vi "Basic Test Compile 2, Proof of Concept.vi"() -> ()   [LabVIEW 2009]
uses:
  Motor Control Global.vi
  <vilib>/Platform/TimedLoop/XDataNode/XDataNode.xnode
  <vilib>/Platform/TimedLoop/XDataNode/loadlvalarms.vi
  <vilib>/Platform/TimedLoop/XDataNode/timing_clust.ctl
  <vilib>/Platform/TimedLoop/XDataNode/nitl_modes.ctl
  <vilib>/Platform/TimedLoop/XDataNode/wakeup.ctl
  <vilib>/Platform/TimedLoop/XDataNode/XDNodeRunTimeDep.lvlib
panel:
  in  "Input A 2":fxp<+/-,18,1>
  out "13 Timed out":bool
  out "Timed out":bool
  out "12 Timed out":bool
  out "Tick Count Differencce":u32
  out "Tick Count(Ticks) 2":u32 caption="Tick Count(Ticks)"
  out "Tick Count(Ticks)":u32
  in  "Single Cycle":bool
  out "Multiplication Result":fxp<+/-,18,1> format="%.18g"
  out "i 3":i32
  out "i 2":i32
  out "i 1":i32
  out "in wait":bool=TRUE
  in  "Restart":bool
  in  "Input F":fxp<+/-,18,1>
  in  "Input E":fxp<+/-,18,1>
  out "Multiplication Result 8 iterations of madness":fxp<+/-,18,1> format="%.18g"
  in  "Input D":fxp<+/-,18,1>
  in  "Input C":fxp<+/-,18,1>
  out "Multiplication Result C^2^15 * D^2^15":fxp<+/-,18,1> format="%.18g"
  in  "stop":bool
  out "Multiplication Result A^60*B":fxp<+/-,18,1> format="%.18g"
  in  "Input A":fxp<+/-,18,1>
  in  "Input B":fxp<+/-,18,1>
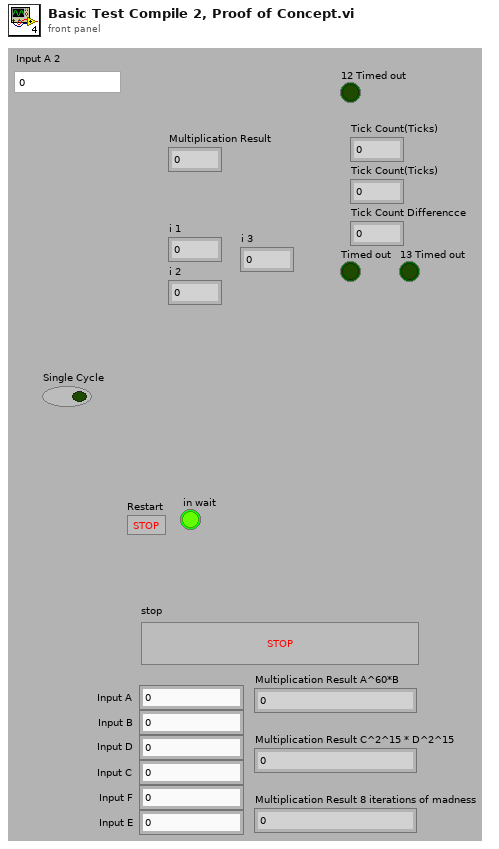
[diagram p1: front panel]
types:
  T1 = typedef "XDNodeRunTimeDep.lvlib/timing_clust.ctl" = cluster{"Expected End [f-1]":u64, "Actual End [f-1]":u64, "Finished Late? [f-1]":bool, "Expected End [i-1]":u64, "Actual End [i-1]":u64, "Finished Late? [i-1]":bool, "Expected Start [i]":u64, "Actual Start [i]":u64, "Expected Start [f]":u64, "Actual Start [f]":u64, "Source Name":string, "Structure Name":string, "Period":i64, "Deadline":i64, "Offset":i64, "Start":i64, "Priority":i32, "Timeout":i32, "Mode":T2, "Wakeup Reason":T3, "Error":errorcluster, "Source Type":string, "Secondary Source Type":string, "Global End Time":u64, "Global Start Time":u64, "Frame Duration":u64, "Iteration Duration":u64, "Assigned CPU":i32, "I/O Scan Engine Mode":u32}
  T2 = typedef "XDNodeRunTimeDep.lvlib/nitl_modes.ctl" = enum32{"No Change", "Process missed periods, maintain original phase", "Discard missed periods, maintain original phase", "Process missed periods, ignore original phase", "Discard missed periods, ignore original phase"}
  T3 = typedef "XDNodeRunTimeDep.lvlib/wakeup.ctl" = enum32{"Normal", "Aborted", "Asynchronous wakeup", "Timing source error", "Timed loop error", "Timeout"}
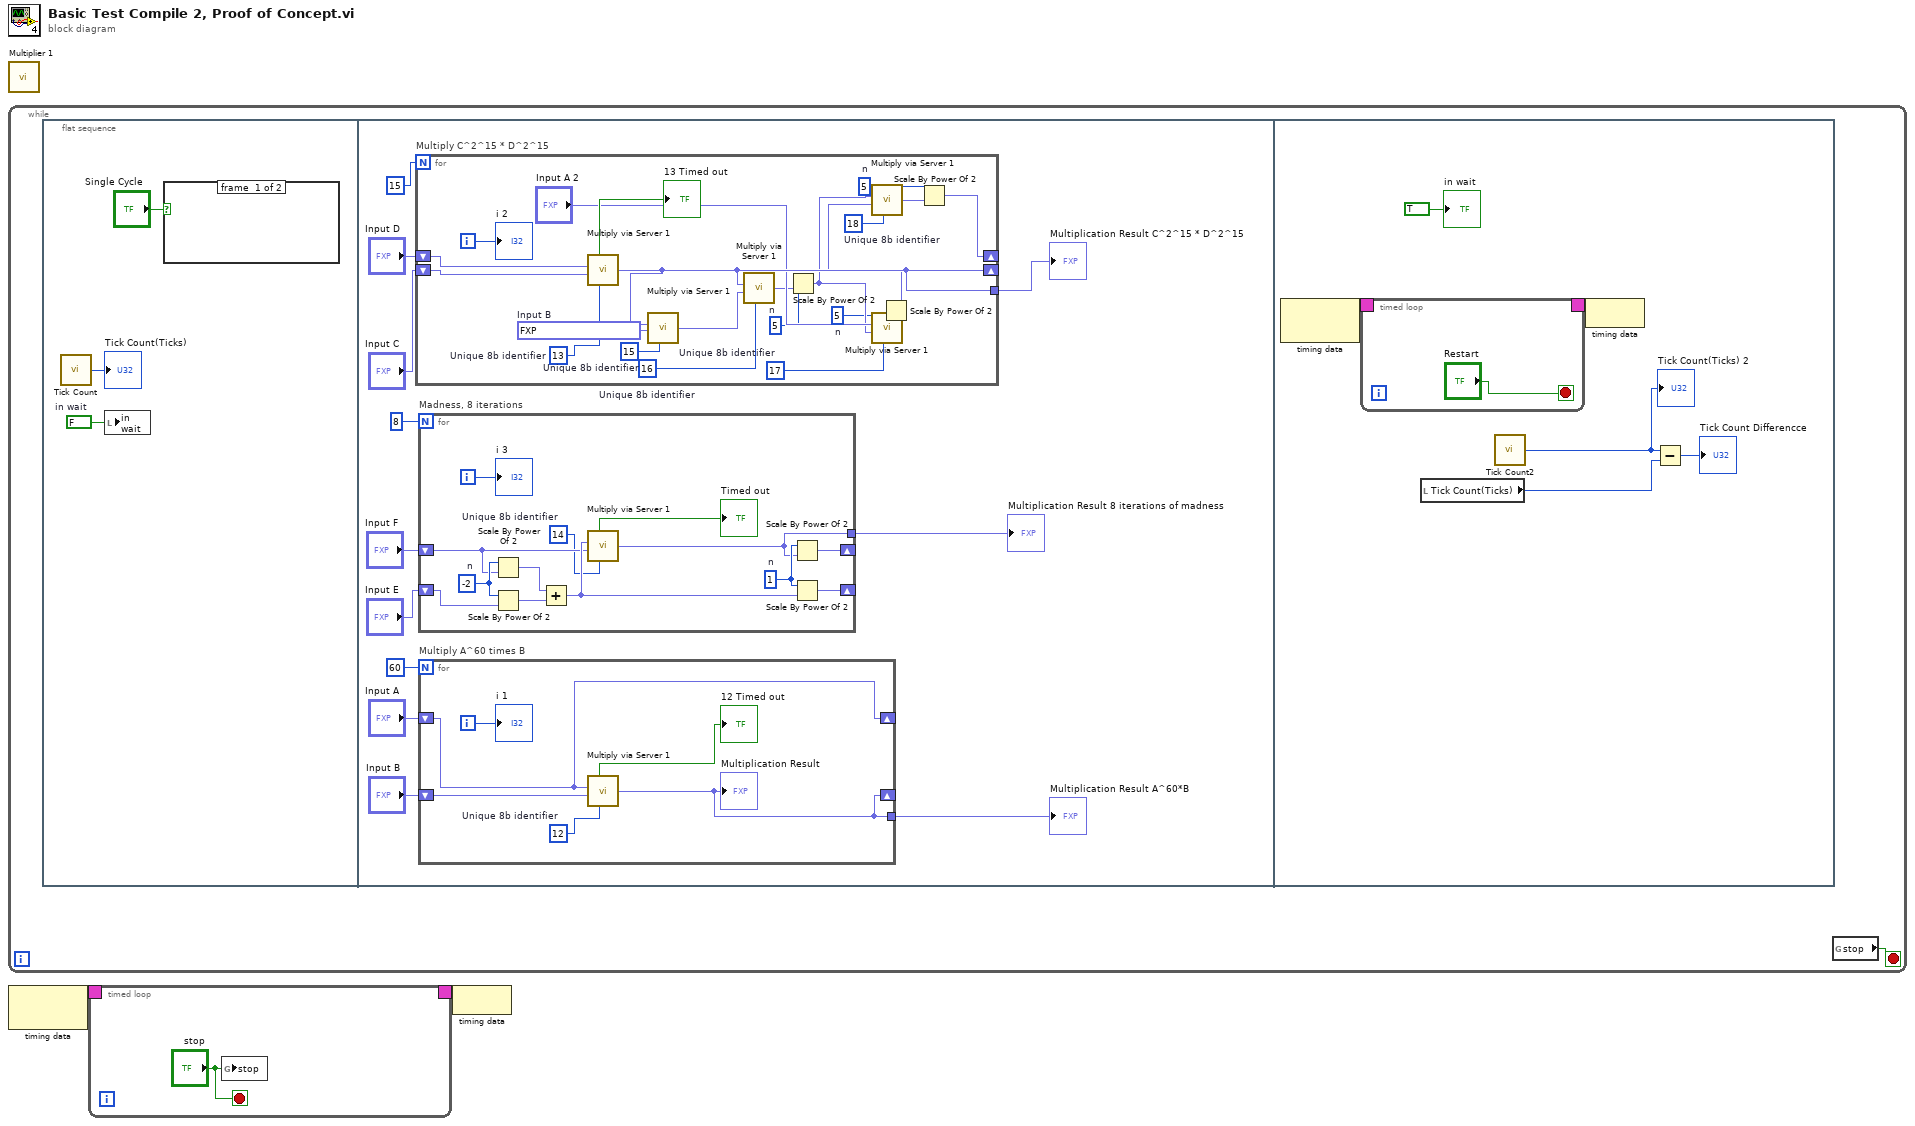
[diagram p0: block diagram]
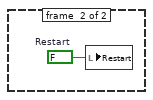
[diagram p2: hidden frame]
diagram:
  n1 = call "Multiplier 1.vi"() -> ()  [unwired: 1 in]
  n2 = while {
    stop <- w3 stop-if-true
    n3 = flat-sequence {
      frame #0 {
        w6 = FALSE  # in wait
        n4 = call "Tick Count"() -> ("Tick Count(Ticks)"=→"Tick Count(Ticks)":u32)
        n5 = local write "in wait"(w6) -> ()
        n6 = case shown="True" "Single Cycle" {
          frame #0 {
          }
          frame #1 {
            w7 = FALSE  # Restart
            n7 = local write "Restart"(w7) -> ()
          }
        }
      }
      frame #1 {
        n8 = for "Multiply C^2^15 * D^2^15" {
          N: 15 -> [_]
          shift-right: [w36] -> _
          shift-left: "Input D" -> [w53]
          shift-right: [w46] -> _
          shift-left: "Input C" -> [w52]
          tunnel: [w46] -> w15
          i -> [w54]
          w33 = 5  # n
          w35 = 5  # n
          w37 = 5  # n
          w43 = u8 18  # Unique 8b identifier
          w44 = u8 17  # Unique 8b identifier
          w45 = u8 16  # Unique 8b identifier
          w48 = u8 15  # Unique 8b identifier
          w49 = fxp<+/-,18,1> 0.7323379516601562  # Input B
          w51 = u8 13  # Unique 8b identifier
          n9 = call "Multiply via Server 1.vi"("Unique 8b identifier"=w51, "Input B"=w52, "Input A"=w53) -> ("Output"=w46:fxp<+/-,18,1>, "Timed out"=→"13 Timed out":bool)  [unwired: 2 in]
          n10 = call "Multiply via Server 1.vi"("Unique 8b identifier"=w48, "Input B"=w49, "Input A"=w46) -> ("Output"=w47:fxp<+/-,18,1>)  [unwired: 2 in, 1 out]
          n11 = call "Multiply via Server 1.vi"("Unique 8b identifier"=w45, "Input B"=w47, "Input A"=w46) -> ("Output"=w41:fxp<+/-,18,1>)  [unwired: 2 in, 1 out]
          n12 = Scale By Power Of 2(n=w37, x=w41) -> (x*2^n=w38:fxp<+/-,18,1>)
          n13 = call "Multiply via Server 1.vi"("Unique 8b identifier"=w44, "Input B"=w38, "Input A"="Input A 2") -> ("Output"=w40:fxp<+/-,18,1>)  [unwired: 2 in, 1 out]
          n14 = Scale By Power Of 2(n=w33, x=w40) -> (x*2^n=w34:fxp<+/-,18,1>)
          n15 = call "Multiply via Server 1.vi"("Unique 8b identifier"=w43, "Input B"=w34, "Input A"=w38) -> ("Output"=w39:fxp<+/-,18,1>)  [unwired: 2 in, 1 out]
          n16 = Scale By Power Of 2(n=w35, x=w39) -> (x*2^n=w36:fxp<+/-,18,1>)
          "i 2" <- w54
        }
        "Multiplication Result C^2^15 * D^2^15" <- w15
        n17 = for "Madness, 8 iterations" {
          N: 8 -> [_]
          shift-right: [w30] -> _
          shift-left: "Input F" -> [w23]
          shift-right: [w29] -> _
          shift-left: "Input E" -> [w32]
          tunnel: [w22] -> w8
          i -> [w31]
          w28 = 1  # n
          w27 = -2  # n
          w21 = u8 14  # Unique 8b identifier
          n18 = Scale By Power Of 2(n=w27, x=w23) -> (x*2^n=w26:fxp<+/-,18,1>)
          n19 = Scale By Power Of 2(n=w27, x=w32) -> (x*2^n=w25:fxp<+/-,18,1>)
          n20 = Add(x=w26, y=w25) -> (x+y=w24:fxp<+/-,18,1>)
          n21 = call "Multiply via Server 1.vi"("Unique 8b identifier"=w21, "Input B"=w23, "Input A"=w24) -> ("Output"=w22:fxp<+/-,18,1>, "Timed out"=→"Timed out":bool)  [unwired: 2 in]
          n22 = Scale By Power Of 2(n=w28, x=w22) -> (x*2^n=w30:fxp<+/-,18,1>)
          n23 = Scale By Power Of 2(n=w28, x=w24) -> (x*2^n=w29:fxp<+/-,18,1>)
          "i 3" <- w31
        }
        "Multiplication Result 8 iterations of madness" <- w8
        n24 = for "Multiply A^60 times B" {
          N: 60 -> [_]
          shift-right: [w59] -> _
          shift-left: "Input A" -> [w59]
          shift-right: [w56] -> _
          shift-left: "Input B" -> [w58]
          tunnel: [w56] -> w16
          i -> [w60]
          w57 = u8 12  # Unique 8b identifier
          n25 = call "Multiply via Server 1.vi"("Unique 8b identifier"=w57, "Input B"=w58, "Input A"=w59) -> ("Output"=w56:fxp<+/-,18,1>, "Timed out"=→"12 Timed out":bool)  [unwired: 2 in]
          "Multiplication Result" <- w56
          "i 1" <- w60
        }
        "Multiplication Result A^60*B" <- w16
      }
      frame #2 {
        n26 = node-c288() -> (w65:T1)  [unwired: 1 in]
        n27 = timed-loop {
          timing: w65 -> [_]
          timing-out: [_] -> w64
          stop <- "Restart" stop-if-true
        }
        n28 = local read "Tick Count(Ticks)"() -> (w66:u32)
        n29 = call "Tick Count2"() -> ("Tick Count(Ticks)"=w62:u32)
        "Tick Count(Ticks) 2" <- w62
        n30 = node-c288(w64) -> ()
        n31 = Subtract(x=w62, y=w66) -> (x-y=→"Tick Count Differencce":u32)
        "in wait" <- TRUE
      }
    }
    n32 = global read "Motor Control Global.vi" "stop"() -> (w3:bool)
  }
  n33 = node-c288() -> (w2:T1)  [unwired: 1 in]
  n34 = timed-loop {
    timing: w2 -> [_]
    timing-out: [_] -> w1
    stop <- "stop" stop-if-true
    n35 = global write "Motor Control Global.vi" "stop"("stop") -> ()
  }
  n36 = node-c288(w1) -> ()
